vi "DAQControl.vi"() -> ()   [LabVIEW 2011]
panel:
  out "AIN data":dbl
  out "Offsets":dbl[](array[numeric])
  out "Gains":dbl[](array[numeric])
  out "connected to device":bool
  in  "Quit":bool
  in  "LED 2":i8=1 min=1 max=3 step=1
  in  "?":bool
  in  "VISA resourceINPUT":refnum<visa-resource-name>
  in  "?":T1(tab)
  in  "START":bool
  in  "stop":bool
  in  "Rate (ms)":dbl=500.0 min=1.0 max=65535.0 step=1.0 format="%#_5g"
  in  "Range":string(combo)="1"
  in  "Ch-":string(combo)="0"
  in  "Ch+":string(combo)="8"
  out "Waveform Chart":dbl(graph)
  in  "Output (Volts) 2":sgl(slide) caption="Output (Volts)" min=-4.096 max=4.096 step=0.001 scale=-4.096..4.096 scale format="%#.2f"
  in  "?":bool
  out "Port Direction:":string
  out "Port State:":string
  in  "all inputs":bool
  in  "all outputs":bool
  in  "d6 set":enum32{"D6", "Radio Selection 2"}(radio)
  in  "d5 set":enum32{"D5", "Radio Selection 2"}(radio)
  in  "d4 set":enum32{"D4", "Radio Selection 2"}(radio)
  in  "d3 set":enum32{"D3", "Radio Selection 2"}(radio)
  in  "d2 set":enum32{"D2", "Radio Selection 2"}(radio)
  in  "D1 set":enum32{"D1", "Radio Selection 2"}(radio)
  in  "?":bool
  out "D1 2":bool caption="D1"
  in  "D1":bool
  out "D3 2":bool caption="D3"
  in  "D3":bool
  in  "D4 2":bool caption="D4"
  out "D5 2":bool caption="D5"
  in  "D6 2":bool caption="D6"
  out "D2":bool
  out "D4":bool
  out "D6":bool
  in  "D2":bool
  in  "D5":bool
  in  "Enable":bool
  in  "Duty (0-1023):":dbl
  in  "Period (us):":dbl
  out "Pulse Length (ms):":dbl
  in  "Boolean 3":bool
  in  "Radio Buttons 9":enum32{"Radio Selection 1", "Radio Selection 2"}(radio)
  out "Count:":i16
  in  "Radio Buttons":T2(radio)
  in  "Update":bool
  in  "Radio Buttons 8":enum32{"Radio Selection 1", "Radio Selection 2"}(radio)
  # "Output"
  # "Input"
  # "[1            6]"
  # "[1            6]"
  # "D1"
  # "D2"
  # "D3"
  # "D4"
  # "D5"
  # "D6"
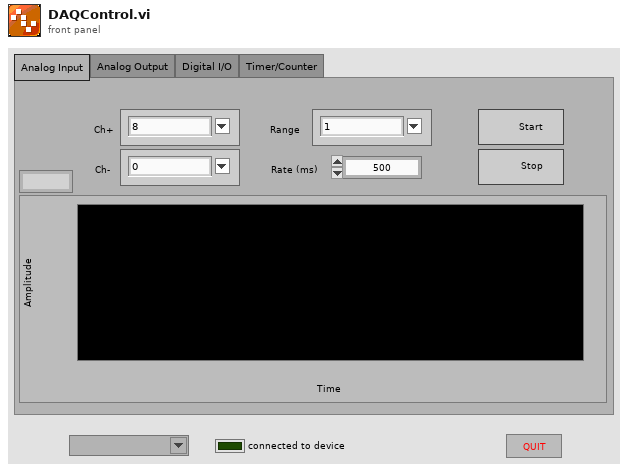
[diagram p1: front panel]
types:
  T1 = enum32{"Analog Input", "Analog Output", "Digital I/O", "Timer/Counter"}
  T2 = enum32{"Radio Selection 1", "Radio Selection 2", "Radio Selection 3"}
  T3 = enum8{"Enabled", "Disabled", "Disabled and Grayed Out"}
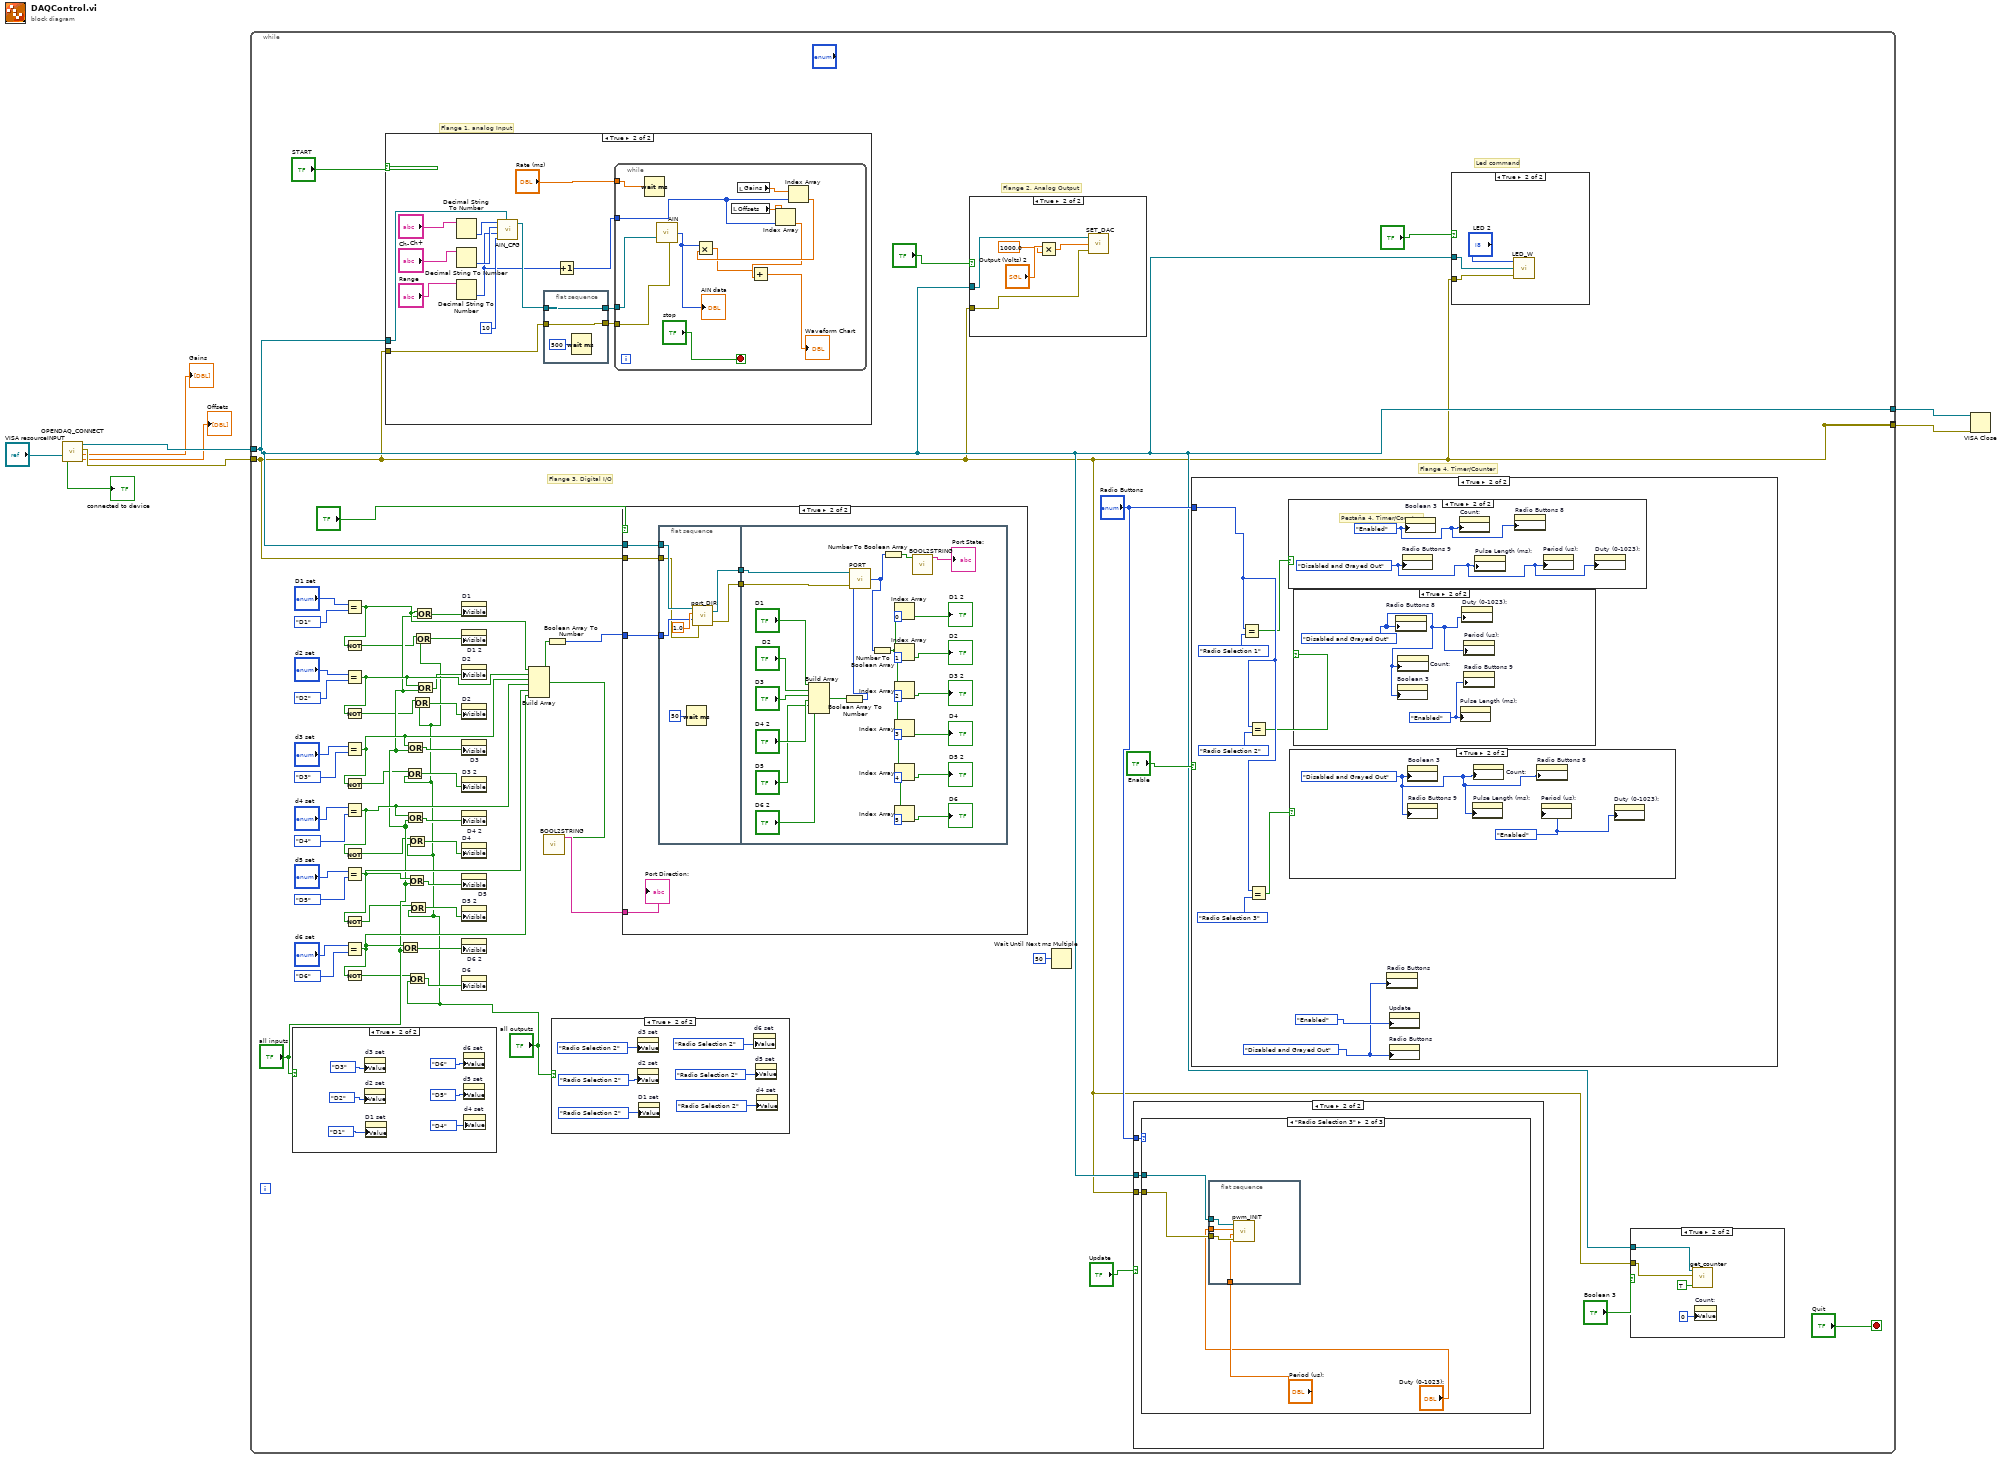
[diagram p0: block diagram]
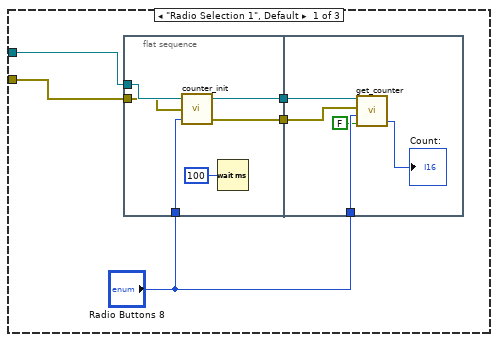
[diagram p4: hidden frame]
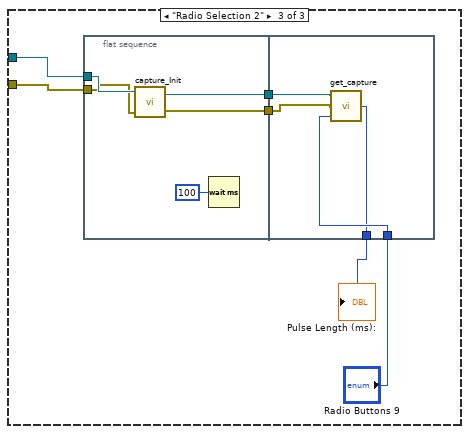
[diagram p5: hidden frame]
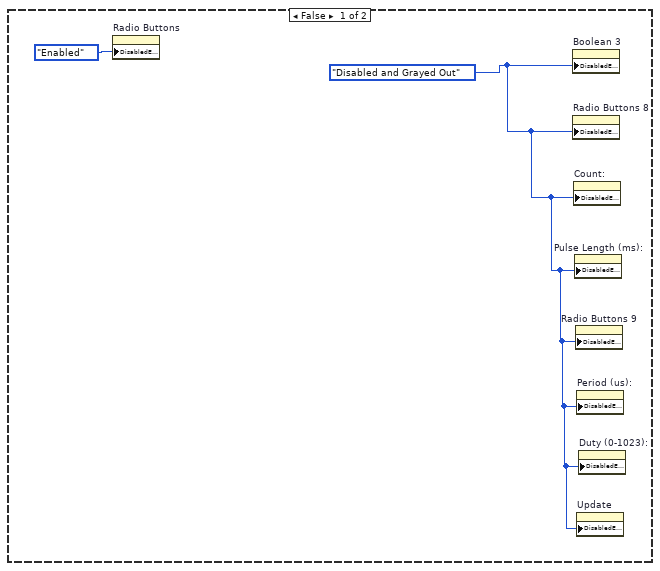
[diagram p6: hidden frame]
diagram:
  n1 = call "OPENDAQ_CONNECT.vi"("VISA resourceINPUT"="VISA resourceINPUT") -> ("connected to device"=→"connected to device":bool, "VISA resource Salida"=w4:refnum<visa-resource-name>, "error out"=w3:errorcluster, "Gains"=→"Gains":dbl[], "Offsets"=→"Offsets":dbl[])
  n2 = while {
    tunnel: w4 -> [w10]
    tunnel: w3 -> [w9]
    tunnel: [w10] -> w8
    tunnel: [w9] -> _
    tunnel: [w9] -> w7
    stop <- "Quit" stop-if-true
    # "Flange 4, Timer/Counter"
    # "Flange 1, analog Input"
    # "Flange 3, Digital I/O"
    # "Flange 2, Analog Output"
    # "Led command"
    n3 = case shown="True" "all inputs" {
      frame False {
      }
      frame True {
        n4 = property on="d3 set" class="RadioBtnsControl (strict)"("Value"=enum32{"D3", "Radio Selection 2"}."D3" ("d3 set")) -> ()  [unwired: 2 in, 2 out]
        n5 = property on="d2 set" class="RadioBtnsControl (strict)"("Value"=enum32{"D2", "Radio Selection 2"}."D2" ("d2 set")) -> ()  [unwired: 2 in, 2 out]
        n6 = property on="D1 set" class="RadioBtnsControl (strict)"("Value"=enum32{"D1", "Radio Selection 2"}."D1" ("D1 set")) -> ()  [unwired: 2 in, 2 out]
        n7 = property on="d6 set" class="RadioBtnsControl (strict)"("Value"=enum32{"D6", "Radio Selection 2"}."D6" ("d6 set")) -> ()  [unwired: 2 in, 2 out]
        n8 = property on="d5 set" class="RadioBtnsControl (strict)"("Value"=enum32{"D5", "Radio Selection 2"}."D5" ("d5 set")) -> ()  [unwired: 2 in, 2 out]
        n9 = property on="d4 set" class="RadioBtnsControl (strict)"("Value"=enum32{"D4", "Radio Selection 2"}."D4" ("d4 set")) -> ()  [unwired: 2 in, 2 out]
      }
    }
    n10 = Equal?(x="D1 set", y=enum32{"D1", "Radio Selection 2"}."D1") -> (x = y?=w30:bool)
    n11 = Not(x=w30) -> (.not. x?=w17:bool)
    n12 = Equal?(x="d2 set", y=enum32{"D2", "Radio Selection 2"}."D2") -> (x = y?=w32:bool)
    n13 = Not(x=w32) -> (.not. x?=w19:bool)
    n14 = Equal?(x="d3 set", y=enum32{"D3", "Radio Selection 2"}."D3") -> (x = y?=w34:bool)
    n15 = Not(x=w34) -> (.not. x?=w24:bool)
    n16 = Equal?(x="d4 set", y=enum32{"D4", "Radio Selection 2"}."D4") -> (x = y?=w36:bool)
    n17 = Not(x=w36) -> (.not. x?=w25:bool)
    n18 = Equal?(x="d5 set", y=enum32{"D5", "Radio Selection 2"}."D5") -> (x = y?=w38:bool)
    n19 = Not(x=w38) -> (.not. x?=w26:bool)
    n20 = Equal?(x="d6 set", y=enum32{"D6", "Radio Selection 2"}."D6") -> (x = y?=w40:bool)
    n21 = Not(x=w40) -> (.not. x?=w27:bool)
    n22 = case shown="True" "START" {
      tunnel: w10 -> [_ w146]
      tunnel: w9 -> [_ w140]
      frame False {
      }
      frame True {
        n23 = Decimal String To Number(string="Ch+") -> (number=w144:i32)  [unwired: 2 in, 1 out]
        n24 = Decimal String To Number(string="Ch-") -> (number=w145:i32)  [unwired: 2 in, 1 out]
        n25 = Decimal String To Number(string="Range") -> (number=w138:i32)  [unwired: 2 in, 1 out]
        n26 = call "AIN_CFG.vi"("P-Channel"=w144, "VISA resource name"=w146, "N-Channel"=w145, "Gain"=w138, "nsamples"=i8 10) -> ("VISA resource Salida"=w142:refnum<visa-resource-name>)  [unwired: 1 in, 2 out]
        n27 = flat-sequence {
          tunnel: w142 -> [w153]
          tunnel: [w153] -> w141
          tunnel: [w152] -> w139
          tunnel: w140 -> [w152]
          frame #0 {
            n28 = Wait (ms)(milliseconds to wait=u32 500) -> ()  [unwired: 1 out]
          }
        }
        n29 = Increment(x=w138) -> (x+1=w137:i32)
        n30 = while {
          tunnel: "Rate (ms)" -> [w164]
          tunnel: w141 -> [w163]
          tunnel: w139 -> [w162]
          tunnel: w137 -> [w159]
          stop <- "stop" stop-if-true
          n31 = Wait (ms)(milliseconds to wait=w164) -> ()  [unwired: 1 out]
          n32 = call "AIN.vi"("VISA resource name"=w163, "error in (no error)"=w162) -> ("AIN data"=w158:i16)  [unwired: 2 out]
          "AIN data" <- w158
          n33 = local read "Offsets"() -> (w160:dbl[])
          n34 = local read "Gains"() -> (w161:dbl[])
          n35 = Index Array(array=w160, index=w159) -> (element=w156:dbl)
          n36 = Index Array(array=w161, index=w159) -> (element=w157:dbl)
          n37 = Multiply(x=w158, y=w157) -> (x*y=w155:dbl)
          n38 = Add(x=w155, y=w156) -> (x+y=→"Waveform Chart":dbl)
        }
      }
    }
    n39 = Or(x=w40, y="all inputs") -> (x .or. y?=w39:bool)
    n40 = Or(x=w24, y="all outputs") -> (x .or. y?=w23:bool)
    n41 = Or(x=w34, y="all inputs") -> (x .or. y?=w33:bool)
    n42 = Or(x=w36, y="all inputs") -> (x .or. y?=w35:bool)
    n43 = Or(x=w38, y="all inputs") -> (x .or. y?=w37:bool)
    n44 = Or(x=w25, y="all outputs") -> (x .or. y?=w22:bool)
    n45 = Or(x=w27, y="all outputs") -> (x .or. y?=w20:bool)
    n46 = Or(x=w26, y="all outputs") -> (x .or. y?=w21:bool)
    n47 = Or(x=w19, y="all outputs") -> (x .or. y?=w18:bool)
    n48 = Or(x=w17, y="all outputs") -> (x .or. y?=w16:bool)
    n49 = Or(x=w30, y="all inputs") -> (x .or. y?=w28:bool)
    n50 = Or(x=w32, y="all inputs") -> (x .or. y?=w31:bool)
    n51 = property on="D1" class="Bool (strict)"("Visible"=w28) -> ()  [unwired: 2 in, 2 out]
    n52 = property on="D1 2" class="Bool (strict)"("Visible"=w16) -> ()  [unwired: 2 in, 2 out]
    n53 = property on="D2" class="Bool (strict)"("Visible"=w31) -> ()  [unwired: 2 in, 2 out]
    n54 = property on="D2" class="Bool (strict)"("Visible"=w18) -> ()  [unwired: 2 in, 2 out]
    n55 = property on="D3" class="Bool (strict)"("Visible"=w33) -> ()  [unwired: 2 in, 2 out]
    n56 = property on="D3 2" class="Bool (strict)"("Visible"=w23) -> ()  [unwired: 2 in, 2 out]
    n57 = property on="D4 2" class="Bool (strict)"("Visible"=w35) -> ()  [unwired: 2 in, 2 out]
    n58 = property on="D4" class="Bool (strict)"("Visible"=w22) -> ()  [unwired: 2 in, 2 out]
    n59 = property on="D5" class="Bool (strict)"("Visible"=w37) -> ()  [unwired: 2 in, 2 out]
    n60 = property on="D5 2" class="Bool (strict)"("Visible"=w21) -> ()  [unwired: 2 in, 2 out]
    n61 = property on="D6 2" class="Bool (strict)"("Visible"=w39) -> ()  [unwired: 2 in, 2 out]
    n62 = property on="D6" class="Bool (strict)"("Visible"=w20) -> ()  [unwired: 2 in, 2 out]
    n63 = Build Array(w30, w32, w34, w36, w38, w40) -> (w41:bool[])
    n64 = call "BOOL2STRING.vi"("Array"=w41) -> ("String"=w42:string)  [unwired: 10 in]
    n65 = Boolean Array To Number(Boolean array=w41) -> (number=w43:u32)
    n66 = case shown="True" "all outputs" {
      frame False {
      }
      frame True {
        n67 = property on="d3 set" class="RadioBtnsControl (strict)"("Value"=enum32{"D3", "Radio Selection 2"}."Radio Selection 2" ("d3 set")) -> ()  [unwired: 2 in, 2 out]
        n68 = property on="d2 set" class="RadioBtnsControl (strict)"("Value"=enum32{"D2", "Radio Selection 2"}."Radio Selection 2" ("d2 set")) -> ()  [unwired: 2 in, 2 out]
        n69 = property on="D1 set" class="RadioBtnsControl (strict)"("Value"=enum32{"D1", "Radio Selection 2"}."Radio Selection 2" ("D1 set")) -> ()  [unwired: 2 in, 2 out]
        n70 = property on="d6 set" class="RadioBtnsControl (strict)"("Value"=enum32{"D6", "Radio Selection 2"}."Radio Selection 2" ("d6 set")) -> ()  [unwired: 2 in, 2 out]
        n71 = property on="d5 set" class="RadioBtnsControl (strict)"("Value"=enum32{"D5", "Radio Selection 2"}."Radio Selection 2" ("d5 set")) -> ()  [unwired: 2 in, 2 out]
        n72 = property on="d4 set" class="RadioBtnsControl (strict)"("Value"=enum32{"D4", "Radio Selection 2"}."Radio Selection 2" ("d4 set")) -> ()  [unwired: 2 in, 2 out]
      }
    }
    n73 = case shown="True" "?" {
      tunnel: w9 -> [_ w171]
      tunnel: w10 -> [_ w170]
      tunnel: w43 -> [_ w167]
      tunnel: w42 -> [_ w166]
      frame False {
      }
      frame True {
        n74 = flat-sequence {
          tunnel: w171 -> [w172]
          tunnel: w170 -> [w173]
          tunnel: [w177] -> w169
          tunnel: [w176] -> w168
          tunnel: w167 -> [w175]
          tunnel: w169 -> [w204]
          tunnel: w168 -> [w203]
          frame #0 {
            n75 = Wait (ms)(milliseconds to wait=u32 50) -> ()  [unwired: 1 out]
            n76 = call "port_DIR.vi"("error in (no error)"=w172, "PIOs directions"=w175, "read/write"=1.0 ("Seleccion canal"), "VISA resource Input"=w173) -> ("error out"=w176:errorcluster, "VISA resource name out"=w177:refnum<visa-resource-name>)
          }
          frame #1 {
            n77 = Build Array("D1", "D2", "D3", "D4 2", "D5", "D6 2") -> (w202:bool[])
            n78 = Boolean Array To Number(Boolean array=w202) -> (number=w201:u32)
            n79 = call "PORT.vi"("error INPUT"=w203, "PIOs output"=w201, "VISA resource Input"=w204) -> ("Value"=w181:u8)  [unwired: 2 out]
            n80 = Number To Boolean Array(number=w181) -> (Boolean array=w194:bool[])
            n81 = Number To Boolean Array(number=w181) -> (Boolean array=w180:bool[])
            n82 = Index Array(array=w194, index=0) -> (element=→"D1 2":bool)
            n83 = Index Array(array=w194, index=1) -> (element=→"D2":bool)
            n84 = Index Array(array=w194, index=2) -> (element=→"D3 2":bool)
            n85 = Index Array(array=w194, index=3) -> (element=→"D4":bool)
            n86 = Index Array(array=w194, index=4) -> (element=→"D5 2":bool)
            n87 = Index Array(array=w194, index=5) -> (element=→"D6":bool)
            n88 = call "BOOL2STRING.vi"("Array"=w180) -> ("String"=→"Port State:":string)  [unwired: 10 in]
          }
        }
        "Port Direction:" <- w166
      }
    }
    n89 = case shown="True" "?" {
      tunnel: w10 -> [_ w212]
      tunnel: w9 -> [_ w211]
      frame False {
      }
      frame True {
        n90 = Multiply(x="Output (Volts) 2", y=sgl 1000.0) -> (x*y=w208:sgl)
        n91 = call "SET_DAC.vi"("error in (no error)"=w211, "Input"=w208, "VISA resource Input"=w212) -> ()  [unwired: 2 out]
      }
    }
    n92 = Wait Until Next ms Multiple(millisecond multiple=u32 50) -> ()  [unwired: 1 out]
    n93 = case shown="True" "Update" {
      tunnel: "Radio Buttons" -> [_ w68]
      tunnel: w10 -> [_ w67]
      tunnel: w9 -> [_ w66]
      frame False {
      }
      frame True {
        n94 = case shown="\"Radio Selection 3\"" w68 {
          tunnel: w67 -> [w73 w88 w98]
          tunnel: w66 -> [w72 w87 w97]
          frame "Radio Selection 1", Default {
            n95 = flat-sequence {
              tunnel: w73 -> [w79]
              tunnel: w72 -> [w78]
              tunnel: [w77] -> w71
              tunnel: [w76] -> w70
              tunnel: "Radio Buttons 8" -> [w75]
              tunnel: w71 -> [w84]
              tunnel: w70 -> [w83]
              tunnel: "Radio Buttons 8" -> [w82]
              frame #0 {
                n96 = call "counter_init.vi"("OptionEdge"=w75, "error in (no error)"=w78, "VISA resource name"=w79) -> ("error out"=w76:errorcluster, "VISA resource Salida"=w77:refnum<visa-resource-name>)  [unwired: 1 out]
                n97 = Wait (ms)(milliseconds to wait=u32 100) -> ()  [unwired: 1 out]
              }
              frame #1 {
                n98 = call "get_counter.vi"("reset"=FALSE, "Option Edge"=w82, "error in (no error)"=w83, "VISA resource name"=w84) -> ("count"=→"Count:":u8)  [unwired: 2 out]
              }
            }
          }
          frame "Radio Selection 3" {
            n99 = flat-sequence {
              tunnel: w88 -> [w92]
              tunnel: w87 -> [w91]
              tunnel: "Period (us):" -> [w90]
              tunnel: "Duty (0-1023):" -> [w89]
              frame #0 {
                n100 = call "pwm_INIT.vi"("error in (no error)"=w91, "Period"=w90, "Duty"=w89, "VISA resource name"=w92) -> ()  [unwired: 2 out]
              }
            }
          }
          frame "Radio Selection 2" {
            n101 = flat-sequence {
              tunnel: w98 -> [w103]
              tunnel: w97 -> [w102]
              tunnel: [w101] -> w96
              tunnel: [w100] -> w95
              tunnel: w96 -> [w107]
              tunnel: w95 -> [w106]
              tunnel: "Radio Buttons 9" -> [w105]
              tunnel: [w104] -> w93
              frame #0 {
                n102 = call "capture_Init.vi"("error in (no error)"=w102, "VISA resource name"=w103) -> ("error out"=w100:errorcluster, "VISA resource Salida"=w101:refnum<visa-resource-name>)  [unwired: 1 in]
                n103 = Wait (ms)(milliseconds to wait=u32 100) -> ()  [unwired: 1 out]
              }
              frame #1 {
                n104 = call "get_capture.vi"("Option Edge"=w105, "error in (no error)"=w106, "VISA resource name"=w107) -> ("(hi.lo) Period"=w104:i16)  [unwired: 2 out]
              }
            }
            "Pulse Length (ms):" <- w93
          }
        }
      }
    }
    n105 = case shown="True" "Enable" {
      tunnel: "Radio Buttons" -> [_ w118]
      frame False {
        w108 = T3."Disabled and Grayed Out" ("Disabled")
        n106 = property on="Radio Buttons" class="RadioBtnsControl (strict)"("DisabledEnum"=T3."Enabled" ("Disabled")) -> ()  [unwired: 2 in, 2 out]
        n107 = property on="Boolean 3" class="Bool"("DisabledEnum"=w108) -> ()  [unwired: 2 in, 2 out]
        n108 = property on="Radio Buttons 8" class="RadioBtnsControl (strict)"("DisabledEnum"=w108) -> ()  [unwired: 2 in, 2 out]
        n109 = property on="Count:" class="DigNum (strict)"("DisabledEnum"=w108) -> ()  [unwired: 2 in, 2 out]
        n110 = property on="Pulse Length (ms):" class="DigNum (strict)"("DisabledEnum"=w108) -> ()  [unwired: 2 in, 2 out]
        n111 = property on="Radio Buttons 9" class="RadioBtnsControl (strict)"("DisabledEnum"=w108) -> ()  [unwired: 2 in, 2 out]
        n112 = property on="Period (us):" class="DigNum (strict)"("DisabledEnum"=w108) -> ()  [unwired: 2 in, 2 out]
        n113 = property on="Update" class="Bool"("DisabledEnum"=w108) -> ()  [unwired: 2 in, 2 out]
        n114 = property on="Duty (0-1023):" class="DigNum (strict)"("DisabledEnum"=w108) -> ()  [unwired: 2 in, 2 out]
      }
      frame True {
        w110 = T3."Disabled and Grayed Out" ("Disabled")
        # "Pestaña 4, Timer/Counter"
        n115 = Equal?(x=w118, y=T2."Radio Selection 1") -> (x = y?=w113:bool)
        n116 = Equal?(x=w118, y=T2."Radio Selection 2") -> (x = y?=w112:bool)
        n117 = Equal?(x=w118, y=T2."Radio Selection 3") -> (x = y?=w114:bool)
        n118 = case shown="True" w113 {
          frame False {
          }
          frame True {
            w121 = T3."Disabled and Grayed Out" ("Disabled")
            w122 = T3."Enabled" ("Disabled")
            n119 = property on="Radio Buttons 9" class="RadioBtnsControl (strict)"("DisabledEnum"=w121) -> ()  [unwired: 2 in, 2 out]
            n120 = property on="Boolean 3" class="Bool"("DisabledEnum"=w122) -> ()  [unwired: 2 in, 2 out]
            n121 = property on="Count:" class="DigNum (strict)"("DisabledEnum"=w122) -> ()  [unwired: 2 in, 2 out]
            n122 = property on="Pulse Length (ms):" class="DigNum (strict)"("DisabledEnum"=w121) -> ()  [unwired: 2 in, 2 out]
            n123 = property on="Radio Buttons 8" class="RadioBtnsControl (strict)"("DisabledEnum"=w122) -> ()  [unwired: 2 in, 2 out]
            n124 = property on="Period (us):" class="DigNum (strict)"("DisabledEnum"=w121) -> ()  [unwired: 2 in, 2 out]
            n125 = property on="Duty (0-1023):" class="DigNum (strict)"("DisabledEnum"=w121) -> ()  [unwired: 2 in, 2 out]
          }
        }
        n126 = case shown="True" w114 {
          frame False {
          }
          frame True {
            w119 = T3."Enabled" ("Disabled")
            w120 = T3."Disabled and Grayed Out" ("Disabled")
            n127 = property on="Boolean 3" class="Bool"("DisabledEnum"=w120) -> ()  [unwired: 2 in, 2 out]
            n128 = property on="Radio Buttons 9" class="RadioBtnsControl (strict)"("DisabledEnum"=w120) -> ()  [unwired: 2 in, 2 out]
            n129 = property on="Pulse Length (ms):" class="DigNum (strict)"("DisabledEnum"=w120) -> ()  [unwired: 2 in, 2 out]
            n130 = property on="Count:" class="DigNum (strict)"("DisabledEnum"=w120) -> ()  [unwired: 2 in, 2 out]
            n131 = property on="Radio Buttons 8" class="RadioBtnsControl (strict)"("DisabledEnum"=w120) -> ()  [unwired: 2 in, 2 out]
            n132 = property on="Period (us):" class="DigNum (strict)"("DisabledEnum"=w119) -> ()  [unwired: 2 in, 2 out]
            n133 = property on="Duty (0-1023):" class="DigNum (strict)"("DisabledEnum"=w119) -> ()  [unwired: 2 in, 2 out]
          }
        }
        n134 = case shown="True" w112 {
          frame False {
          }
          frame True {
            w123 = T3."Enabled" ("Disabled")
            w124 = T3."Disabled and Grayed Out" ("Disabled")
            n135 = property on="Radio Buttons 8" class="RadioBtnsControl (strict)"("DisabledEnum"=w124) -> ()  [unwired: 2 in, 2 out]
            n136 = property on="Boolean 3" class="Bool"("DisabledEnum"=w124) -> ()  [unwired: 2 in, 2 out]
            n137 = property on="Count:" class="DigNum (strict)"("DisabledEnum"=w124) -> ()  [unwired: 2 in, 2 out]
            n138 = property on="Pulse Length (ms):" class="DigNum (strict)"("DisabledEnum"=w123) -> ()  [unwired: 2 in, 2 out]
            n139 = property on="Duty (0-1023):" class="DigNum (strict)"("DisabledEnum"=w124) -> ()  [unwired: 2 in, 2 out]
            n140 = property on="Period (us):" class="DigNum (strict)"("DisabledEnum"=w124) -> ()  [unwired: 2 in, 2 out]
            n141 = property on="Radio Buttons 9" class="RadioBtnsControl (strict)"("DisabledEnum"=w123) -> ()  [unwired: 2 in, 2 out]
          }
        }
        n142 = property on="Radio Buttons" class="RadioBtnsControl (strict)"("DisabledEnum"=w110) -> ()  [unwired: 2 in, 2 out]
        n143 = property on="Update" class="Bool"("DisabledEnum"=T3."Enabled" ("Disabled")) -> ()  [unwired: 2 in, 2 out]
        n144 = property on="Radio Buttons" class="RadioBtnsControl (strict)"("DisabledEnum"=w110) -> ()  [unwired: 2 in, 2 out]
      }
    }
    n145 = case shown="True" "?" {
      tunnel: w10 -> [_ w206]
      tunnel: w9 -> [_ w205]
      frame False {
      }
      frame True {
        n146 = call "LED_W.vi"("error INPUT"=w205, "VISA resource Input"=w206, "Option  Led color"="LED 2") -> ()  [unwired: 2 out]
      }
    }
    n147 = case shown="True" "Boolean 3" {
      tunnel: w10 -> [_ w64]
      tunnel: w9 -> [_ w62]
      frame False {
      }
      frame True {
        n148 = call "get_counter.vi"("reset"=TRUE, "error in (no error)"=w62, "VISA resource name"=w64) -> ()  [unwired: 1 in, 3 out]
        n149 = property on="Count:" class="DigNum (strict)"("Value"=i16 0 ("Count:")) -> ()  [unwired: 2 in, 2 out]
      }
    }
  }
  n150 = VISA Close(VISA resource name=w8, error in (no error)=w7) -> ()  [unwired: 1 out]
